vi "Pv gen100 micro1.vi"(0 "FluxStrIn":string, 1 "Numin":i32, 2 "DeltaCellTemp":dbl, 3 "TempMin":dbl, 4 "DeltaCellVoltmV":dbl, 5 "errin":errorcluster, 6 "testlabel":string, 7 "Vmax":dbl, 8 "tab ref":string[][](array[string]), 9 "Vmin":dbl, 10 "ligne à traiter":string[](array[string]), 11 "TempMax":dbl, 12 "step":i32) -> (13 "moulinette":string[](array[string]), 14 "result string":string, 15 "Numout":i32, 19 "errout":errorcluster)   [LabVIEW 2020]
uses:
  SubVi/Param_Stack.vi
  ctrl glo/TestResultGlo.vi
  <vilib>/regexp/Match Regular Expression.xnode
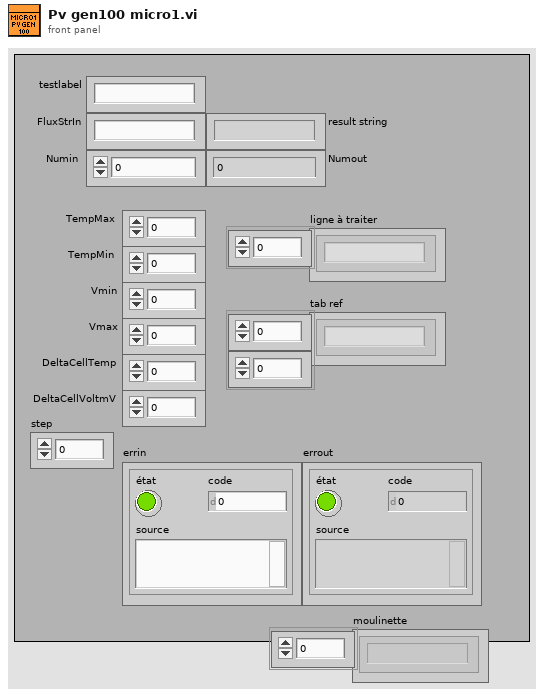
[diagram p1: front panel]
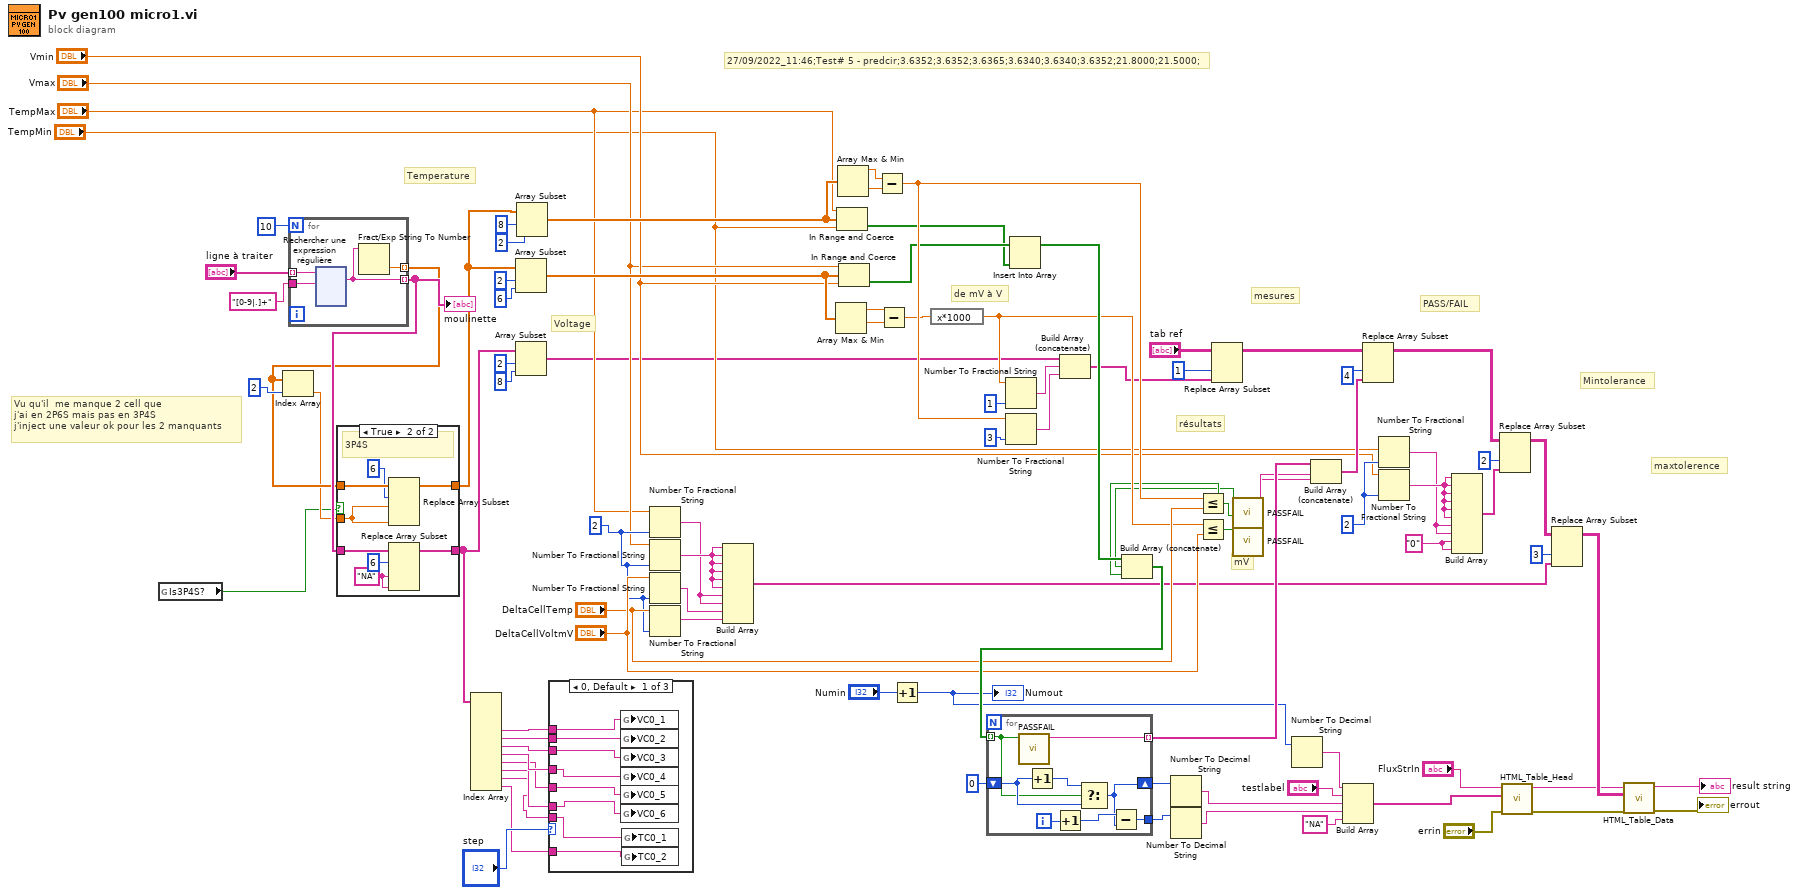
[diagram p0: block diagram]
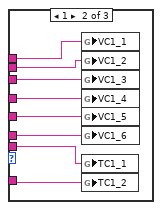
[diagram p2: hidden frame]
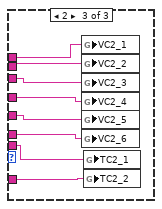
[diagram p3: hidden frame]
diagram:
  w28 = 2
  w29 = 2
  w78 = "0" ("élément")
  # "mV"
  # "maxtolerence"
  # "Mintolerance"
  # "mesures"
  # "Vu qu'il  me manque 2 cell que\nj'ai en 2P6S mais pas en 3P4S\nj'inject une valeur ok pour les 2 manquants"
  # "PASS/FAIL"
  # "résultats"
  # "Voltage"
  # "Temperature"
  # "de mV à V"
  # "27/09/2022_11:46;Test# 5 - predcir;3.6352;3.6352;3.6365;3.6340;3.6340;3.6352;21.8000;21.5000;"
  n1 = global read "Param_Stack.vi" "Is3P4S?"() -> (w11:bool)
  n2 = for {
    N: 10 -> [_]
    tunnel: "ligne à traiter" -> [w97] mode=indexing
    tunnel: "[0-9|.]+" ("expression régulière") -> [w96]
    tunnel: [w95] -> w13 mode=indexing
    tunnel: [w94] -> w22 mode=indexing
    n3 = xnode "Rechercher une expression régulière"("chaîne en entrée"=w97, "expression régulière"=w96) -> ("toute l'expression"=w94:string)  [unwired: 4 in, 4 out]
    n4 = Fract/Exp String To Number(string=w94) -> (number=w95:dbl)  [unwired: 3 in, 1 out]
  }
  "moulinette" <- w22
  n5 = Index Array(array=w13, index=2 ("indice")) -> (element=w12:dbl)
  n6 = case shown="True" w11 {
    tunnel: w13 -> [w213 w221]
    tunnel: [w213 w220] -> w23
    tunnel: w22 -> [w212 w218]
    tunnel: [w212 w217] -> w3
    tunnel: w12 -> [_ w214]
    frame False {
      # "2P6S"
    }
    frame True {
      w215 = "NA" ("nouvel élément/sous-tableau")
      # "3P4S"
      n7 = Replace Array Subset(array=w221, new element #1=w214, index #1=6 ("indice"), new element #2=w214) -> (w220:dbl[])  [unwired: 1 in]
      n8 = Replace Array Subset(array=w218, new element #1=w215, index #1=6 ("indice"), new element #2=w215) -> (w217:string[])  [unwired: 1 in]
    }
  }
  n9 = Index Array(array=w3) -> (element #3=w9:string, element #4=w8:string, element #5=w7:string, element #6=w6:string, element #7=w5:string, element #8=w4:string, element #9=w2:string, element #10=w1:string)  [unwired: 10 in, 2 out]
  n10 = Array Subset(array=w23, index=2 ("indice"), length=6 ("longueur")) -> (w41:dbl[])
  n11 = Array Subset(array=w3, index=2 ("indice"), length=8 ("longueur")) -> (w21:string[])
  n12 = Array Subset(array=w23, index=8 ("indice"), length=2 ("longueur")) -> (w38:dbl[])
  n13 = case shown="0, Default" "step" {
    tunnel: w9 -> [w229 w237 w245]
    tunnel: w8 -> [w228 w236 w244]
    tunnel: w7 -> [w227 w235 w243]
    tunnel: w6 -> [w226 w234 w242]
    tunnel: w5 -> [w225 w233 w241]
    tunnel: w4 -> [w224 w232 w240]
    tunnel: w2 -> [w223 w231 w239]
    tunnel: w1 -> [w222 w230 w238]
    frame 0, Default {
      n14 = global write "TestResultGlo.vi" "VC0_1"(w229) -> ()
      n15 = global write "TestResultGlo.vi" "VC0_2"(w228) -> ()
      n16 = global write "TestResultGlo.vi" "VC0_3"(w227) -> ()
      n17 = global write "TestResultGlo.vi" "VC0_4"(w226) -> ()
      n18 = global write "TestResultGlo.vi" "VC0_5"(w225) -> ()
      n19 = global write "TestResultGlo.vi" "VC0_6"(w224) -> ()
      n20 = global write "TestResultGlo.vi" "TC0_1"(w223) -> ()
      n21 = global write "TestResultGlo.vi" "TC0_2"(w222) -> ()
    }
    frame 1 {
      n22 = global write "TestResultGlo.vi" "VC1_1"(w237) -> ()
      n23 = global write "TestResultGlo.vi" "VC1_2"(w236) -> ()
      n24 = global write "TestResultGlo.vi" "VC1_3"(w235) -> ()
      n25 = global write "TestResultGlo.vi" "VC1_4"(w234) -> ()
      n26 = global write "TestResultGlo.vi" "VC1_5"(w233) -> ()
      n27 = global write "TestResultGlo.vi" "VC1_6"(w232) -> ()
      n28 = global write "TestResultGlo.vi" "TC1_1"(w231) -> ()
      n29 = global write "TestResultGlo.vi" "TC1_2"(w230) -> ()
    }
    frame 2 {
      n30 = global write "TestResultGlo.vi" "VC2_1"(w245) -> ()
      n31 = global write "TestResultGlo.vi" "VC2_2"(w244) -> ()
      n32 = global write "TestResultGlo.vi" "VC2_3"(w243) -> ()
      n33 = global write "TestResultGlo.vi" "VC2_4"(w242) -> ()
      n34 = global write "TestResultGlo.vi" "VC2_5"(w241) -> ()
      n35 = global write "TestResultGlo.vi" "VC2_6"(w240) -> ()
      n36 = global write "TestResultGlo.vi" "TC2_1"(w239) -> ()
      n37 = global write "TestResultGlo.vi" "TC2_2"(w238) -> ()
    }
  }
  n38 = Number To Fractional String(number="TempMax", precision (6)=w28) -> (F-format string=w30:string)  [unwired: 2 in]
  n39 = Number To Fractional String(number="Vmax", precision (6)=w28) -> (F-format string=w31:string)  [unwired: 2 in]
  n40 = Number To Fractional String(number="DeltaCellVoltmV", precision (6)=w28) -> (F-format string=w76:string)  [unwired: 2 in]
  n41 = Number To Fractional String(number="DeltaCellTemp", precision (6)=w28) -> (F-format string=w77:string)  [unwired: 2 in]
  n42 = Build Array(w31, w31, w31, w31, w31, w31, w30, w30, w76, w77) -> (w85:string[])
  n43 = Array Max & Min(array=w41) -> (max value=w72:dbl, min value=w71:dbl)  [unwired: 2 out]
  n44 = In Range and Coerce(upper limit="TempMax", x=w38, lower limit="TempMin") -> (In Range?=w19:bool[])  [unwired: 1 out]
  n45 = Array Max & Min(array=w38) -> (max value=w69:dbl, min value=w70:dbl)  [unwired: 2 out]
  n46 = In Range and Coerce(upper limit="Vmax", x=w41, lower limit="Vmin") -> (In Range?=w20:bool[])  [unwired: 1 out]
  n47 = Subtract(x=w69, y=w70) -> (x-y=w86:dbl)
  n48 = Subtract(x=w72, y=w71) -> (x-y=w74:dbl)
  n49 = Increment(x="Numin") -> (x+1=w60:i32)
  "Numout" <- w60
  n50 = expression code="x*1000"(w74) -> (w87:dbl)
  n51 = Number To Fractional String(number=w87, precision (6)=i16 1 ("précision (6)")) -> (F-format string=w35:string)  [unwired: 2 in]
  n52 = Number To Fractional String(number=w86, precision (6)=i16 3 ("largeur (-)")) -> (F-format string=w34:string)  [unwired: 2 in]
  n53 = Insert Into Array(array=w20, new element=w19) -> (w92:bool[])  [unwired: 1 in]
  n54 = Build Array (concatenate)(w21, w35, w34) -> (w67:string[])
  n55 = Less Or Equal?(x=w86, y="DeltaCellTemp") -> (x <= y?=w18:bool)
  n56 = Less Or Equal?(x=w87, y="DeltaCellVoltmV") -> (x <= y?=w17:bool)
  n57 = Build Array (concatenate)(w92, w17, w18) -> (w93:bool[])
  n58 = for {
    tunnel: w93 -> [w247] mode=indexing
    tunnel: [w246] -> w90 mode=indexing
    shift-right: [w249] -> w62
    shift-left: 0 -> [w252]
    tunnel: [w248] -> w63
    i -> [w251]
    n59 = call <userlib>:"PASSFAIL.vi"("E"=w247) -> ("S"=w246:string)  [unwired: 10 in]
    n60 = Increment(x=w252) -> (x+1=w253:i32)
    n61 = Increment(x=w251) -> (x+1=w250:i32)
    n62 = Select(t=w253, s=w247, f=w252) -> (s? t:f=w249:i32)
    n63 = Subtract(x=w250, y=w249) -> (x-y=w248:i32)
  }
  n64 = Number To Decimal String(number=w62) -> (decimal integer string=w64:string)  [unwired: 1 in]
  n65 = Number To Decimal String(number=w63) -> (decimal integer string=w65:string)  [unwired: 1 in]
  n66 = Replace Array Subset(array="tab ref", new element=w67, index (col)=1 ("indice désactivé (col)")) -> (w47:string[][])  [unwired: 1 in]
  n67 = call <userlib>:"PASSFAIL.vi"("E"=w17) -> ("S"=w15:string)  [unwired: 10 in]
  n68 = call <userlib>:"PASSFAIL.vi"("E"=w18) -> ("S"=w16:string)  [unwired: 10 in]
  n69 = Number To Decimal String(number=w60) -> (decimal integer string=w48:string)  [unwired: 1 in]
  n70 = Build Array (concatenate)(w90, w16, w15) -> (w91:string[])
  n71 = Build Array(w48, "testlabel", w64, w65, "NA" ("élément")) -> (w51:string[])
  n72 = Replace Array Subset(array=w47, new element=w91, index (col)=4 ("indice désactivé (col)")) -> (w79:string[][])  [unwired: 1 in]
  n73 = Number To Fractional String(number="TempMin", precision (6)=w29) -> (F-format string=w32:string)  [unwired: 2 in]
  n74 = Number To Fractional String(number="Vmin", precision (6)=w29) -> (F-format string=w33:string)  [unwired: 2 in]
  n75 = Build Array(w33, w33, w33, w33, w33, w33, w32, w32, w78, w78) -> (w84:string[])
  n76 = Replace Array Subset(array=w79, new element=w84, index (col)=2 ("indice désactivé (col)")) -> (w81:string[][])  [unwired: 1 in]
  n77 = call "HTML_Table_Head.vi"("entrée d'erreur (pas d'erreur)"="errin", "Tableau"=w51, "chaîne en entrée"="FluxStrIn") -> ("sortie d'erreur"=w50:errorcluster, "result string"=w49:string)  [unwired: 7 in]
  n78 = Replace Array Subset(array=w81, new element=w85, index (col)=3 ("indice désactivé (col)")) -> (w80:string[][])  [unwired: 1 in]
  n79 = call "HTML_Table_Data.vi"("entrée d'erreur (pas d'erreur)"=w50, "Tableau"=w80, "chaîne en entrée"=w49) -> ("sortie d'erreur"=→"errout":errorcluster, "result string"=→"result string":string)  [unwired: 7 in]
